vi "OpenLabJackU6.vi"(3 "error in":errorcluster, 4 "Select First Found":bool=TRUE, 5 "Connection Type":u16(ring) items=["USB", "Ethernet"], 6 "U6 Address":string="192.168.1.199") -> (0 "error out":errorcluster, 1 "warning out":errorcluster, 2 "Handle":i32)   [LabVIEW 2021]
panel:
  # "inputs"
  # "outputs"
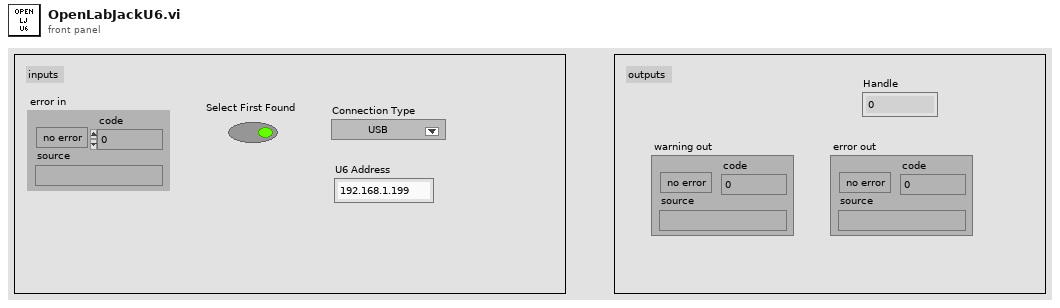
[diagram p1: front panel]
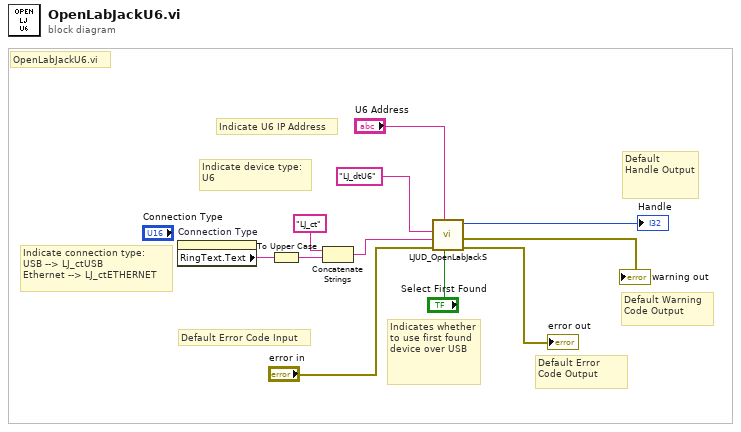
[diagram p0: block diagram]
diagram:
  # "Default Handle Output"
  # "Default Error Code Output"
  # "Default Warning Code Output"
  # "OpenLabJackU6.vi"
  # "Indicate U6 IP Address"
  # "Indicate device type:\nU6"
  # "Indicate connection type:\nUSB --> LJ_ctUSB\nEthernet --> LJ_ctETHERNET"
  # "Indicates whether to use first found device over USB"
  # "Default Error Code Input"
  n1 = property on="Connection Type" class="Ring (strict)"() -> ("RingText.Text"=w1:string)  [unwired: 2 in, 2 out]
  n2 = To Upper Case(1:w1) -> (0:w2:string)
  n3 = Concatenate Strings("LJ_ct" ("string"), w2) -> (w3:string)
  n4 = call <vilib>:"LJUD_OpenLabJackS.vi"("FirstFound"="Select First Found", "Address"="U6 Address", "error in"="error in", "ConnectionType"=w3, "DeviceType"="LJ_dtU6") -> ("error out"=→"error out":errorcluster, "warning out"=→"warning out":errorcluster, "Handle"=→"Handle":i32)  [unwired: 4 in]
